vi "GetHTMLtextforsubsc.vi"(2 "Log":T1, 3 "data":T2) -> (1 "String":string)   [LabVIEW 2012]
uses:
  <userlib>/ROSforLV/ROS/Code/Console/Servers/ServerSubs/requestTopic.ctl
  <userlib>/ROSforLV/ROS/Code/SubVIs/_ROSControl.ctl
  <userlib>/ROSforLV/ROS/Code/SubVIs/_ROSDirection.ctl
  <userlib>/ROSforLV/ROS/Code/Console/Servers/ServerSubs/ROSLog.ctl
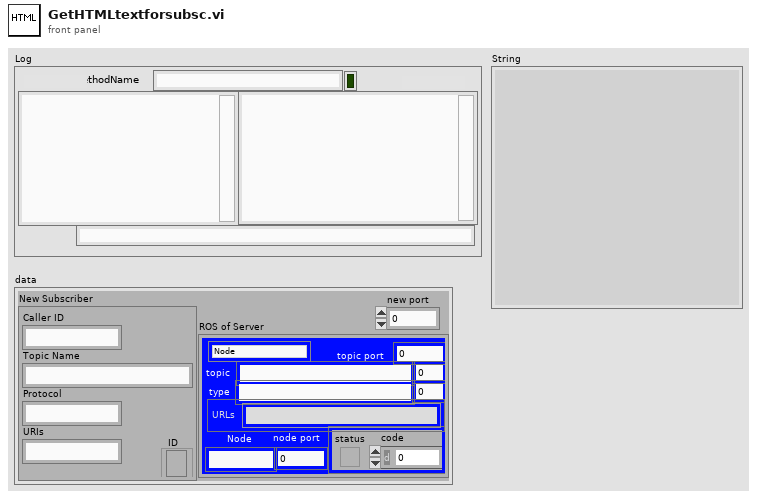
[diagram p1: front panel]
types:
  T1 = typedef "ROSLog.ctl" = cluster{"Sent":string, "Reply":string, "MethodName":string, "success":bool, "Dir1":string, "Dir2":string, "Time Stamp":string, "error":errorcluster, "Preamble":string, "Midamble":string, "Postamble":string}
  T2 = typedef "requestTopic.ctl" = cluster{"New Subscriber":cluster{"Caller ID":string, "Topic Name":string, "Protocol":string, "URIs":string, "ID":refnum<k5>}, "ROS of Server":T3, "new port":u16}
  T3 = typedef "_ROSControl.ctl" = cluster{"topic port":u16, "Node":string, "topic":string, "type":string, "node port":u16, "error ":errorcluster, "Direction":T4, "APIs":string[], "Update (ms)":u16, "write queue":u16}
  T4 = typedef "_ROSDirection.ctl" = enum16{"Node", "Publisher", "Subscriber", "Service Client"}
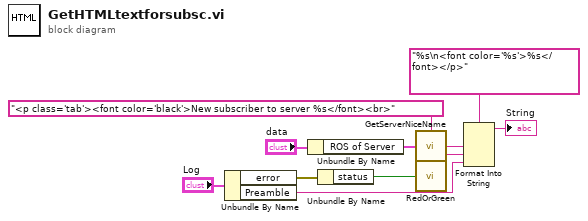
[diagram p0: block diagram]
diagram:
  n1 = Unbundle By Name("Log") -> ("error"=w9:errorcluster, "Preamble"=w1:string)
  n2 = Unbundle By Name("data") -> ("ROS of Server"=w7:T3)
  n3 = Unbundle By Name(w9) -> ("status"=w10:bool)
  n4 = call <userlib>:"GetServerNiceName.vi"("ROS"=w7, "Text to add"="<p class='tab'><font color='black'>New subscriber to server %s</font><br>" ("format string")) -> ("String"=w8:string)
  n5 = call <userlib>:"RedOrGreen.vi"("success"=w10) -> ("color"=w2:string)
  n6 = Format Into String(format string="%s\n<font color='%s'>%s</font></p>", w8, w2, w1) -> (resulting string=→"String":string)  [unwired: 2 in, 1 out]
